vi "Read Previous Item.vi"(8 "error in (no error)":errorcluster, 9 "Wrap? (F)":bool, 11 "StringList Reference":refnum<data-value>) -> (0 "error out":errorcluster, 1 "At Top?":bool, 2 "Item":string, 3 "StringList Reference":refnum<data-value>)   [LabVIEW 2015, in "StringList.lvlib" / "StringList.lvclass"]
uses:
  StringList.lvclass
  StringList.lvclass/StringList.ctl
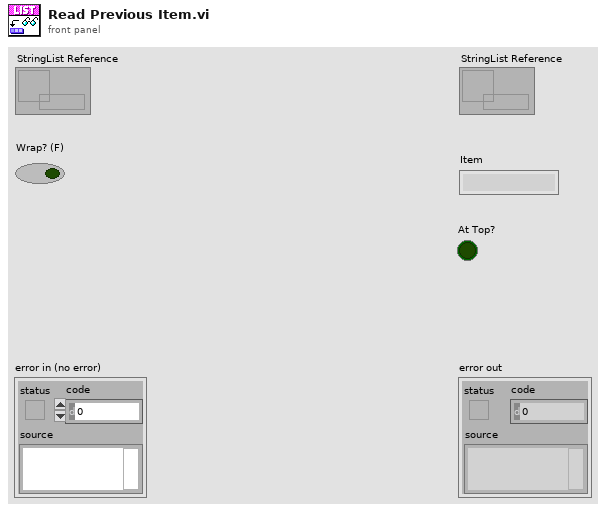
[diagram p1: front panel]
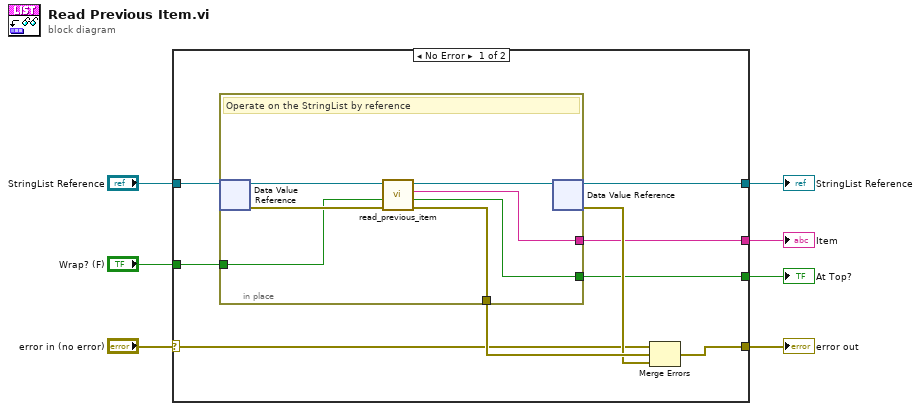
[diagram p0: block diagram]
diagram:
  n1 = case shown="No Error" "error in (no error)" {
    selector: "error in (no error)" -> [w11 w25]
    tunnel: [w16 w25] -> w7
    tunnel: "StringList Reference" -> [w15 w24]
    tunnel: [w14 w24] -> w5
    tunnel: [w10 _] -> w3
    tunnel: "Wrap? (F)" -> [w9 _]
    tunnel: [w8 _] -> w1
    frame No Error {
      n2 = in-place {
        in-place-border: [w20] -> w13
        in-place-border: [w19] -> w10
        in-place-border: w9 -> [w18]
        in-place-border: [w17] -> w8
        # "Operate on the StringList by reference"
        n3 = in-place-dvr #1(w15) -> (w23:refnum<class "StringList.lvclass">, w21:errorcluster)
        n4 = call "read_previous_item.vi"("error in (no error)"=w21, "Wrap? (F)"=w18, "StringList in"=w23) -> ("error out"=w20:errorcluster, "At Top?"=w17:bool, "List Item"=w19:string, "StringList out"=w22:refnum<class "StringList.lvclass">)  [unwired: 5 in]
        n5 = in-place-dvr #1(w22) -> (w14:refnum<data-value>, w12:errorcluster)
      }
      n6 = Merge Errors(w11, w13, w12) -> (w16:errorcluster)
    }
    frame Error {
    }
  }
  "error out" <- w7
  "StringList Reference" <- w5
  "Item" <- w3
  "At Top?" <- w1
